vi "Target.vi"() -> ()   [LabVIEW 2019]
uses:
  <vilib>/rvi/DataTransferAndStorage/Container/Common/niFpgaContainerExecOnDevCompGetState.vi
  <vilib>/rvi/Emulation/niFpgaEmulationIsFPGAContextNoSignature.vi
  <vilib>/rvi/Emulation/niFpgaSctlEmulationGetInTimedLoop.vi
  <vilib>/rvi/errors/niFpgaSetErrorForExecOnDevCompSimple.vi
  <vilib>/rvi/eio/common/nirviEmuReportErrorAndStop.vi
  <vilib>/rvi/DataTransferAndStorage/Container/Common/niFpgaContainerGetUniqueNameForEmu.vi
  <vilib>/rvi/FIFO/Fifo_Resource/nirvififoEmulationSetSize.vi
  <vilib>/rvi/FIFO/Fifo_Resource/nirviFifoEmulationQueueMgr.vi
  <instcachedir>/0/nirviFifoEmulationQueueMgr_E5CAEC123FF24DC58D834DCA3CDAA9B5.lvgen/nirviFifoEmulationQueueMgr_E5CAEC123FF24DC58D834DCA3CDAA9B5_006.vi
  <vilib>/rvi/FIFO/Fifo_Resource/nirvififoEmulationDetermineInputValidOut.vi
  <vilib>/rvi/FIFO/Fifo_Resource/nirvififoEmulationCreateLock.vi
  <vilib>/rvi/Emulation/niFpgaProcessEmulError.vi
  <vilib>/rvi/FIFO/Fifo_Resource/nirvififoEmulationObtainLock.vi
  <vilib>/rvi/FIFO/Fifo_Resource/nirvififoEmulationReleaseLock.vi
  <vilib>/rvi/occurrence/nirviWaitOnOccurrenceBase.vi
  <vilib>/rvi/errors/nirviReportUnexpectedCaseInternalError.vi
  <vilib>/rvi/errors/nirviReportUnexpectedCaseInternalError (U32).vi
  <vilib>/Utility/error.llb/Clear Errors.vi
  <vilib>/rvi/interface/RandomDataEmulation/niFpgaRandomDataHandleErrors.vi
  <vilib>/rvi/DataTransferAndStorage/Container/XNode/niFpgaContainer.xnode
  <vilib>/rvi/FIFO/Fifo_Resource/niFpgaFifoEmulationRefIn.vi
panel:
  out "T5":u32 caption="Tick Count(mSec)"
  out "T4":u32 caption="Tick Count(mSec)"
  out "T3":u32 caption="Tick Count(mSec)"
  out "T2":u32 caption="Tick Count(mSec)"
  out "T1":u32 caption="Tick Count(mSec)"
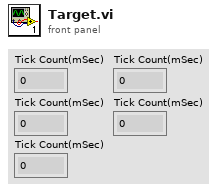
[diagram p1: front panel]
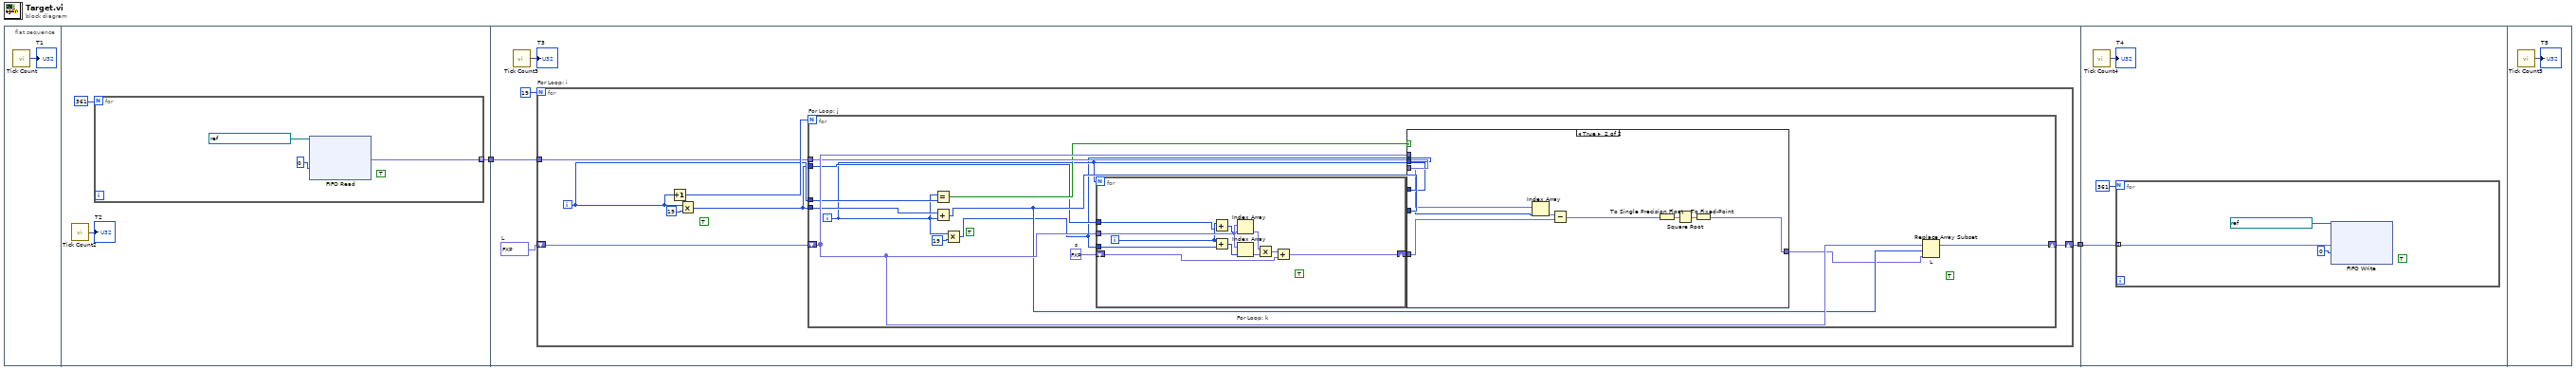
[diagram p0: block diagram]
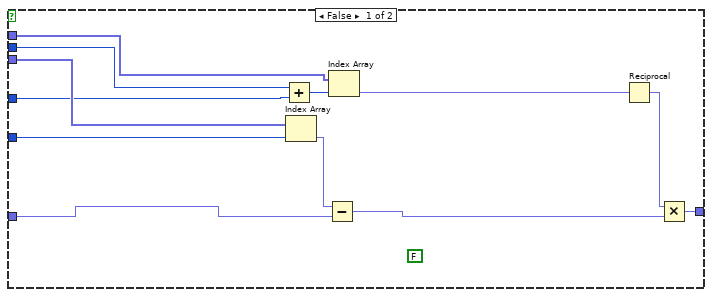
[diagram p2: hidden frame]
diagram:
  n1 = flat-sequence {
    tunnel: [w5] -> w2
    tunnel: w2 -> [w14]
    tunnel: [w13] -> w1
    tunnel: w1 -> [w68]
    frame #0 {
      n2 = call "Tick Count"() -> ("Tick Count(Ticks)"=→"T1":u32)
    }
    frame #1 {
      n3 = call "Tick Count2"() -> ("Tick Count(mSec)"=→"T2":u32)
      n4 = for {
        N: 361 -> [_]
        tunnel: [w9] -> w5 mode=indexing
        (unwired) TRUE
        n5 = xnode ("FIFO Read")("Timeout"=0, "FIFO In"=refnum<k21> "FIFO-host-to-Cholesky") -> ("Element"=w9:fxp<+/-,32,0>)  [unwired: 2 out]
      }
    }
    frame #2 {
      w12 = fxp<+,1,1>[] [0.0, 0.0, 0.0, 0.0, 0.0, 0.0, 0.0, 0.0, 0.0, 0.0, 0.0, 0.0, 0.0, 0.0, 0.0, 0.0, 0.0, 0.0, 0.0, 0.0, 0.0, 0.0, 0.0, 0.0, 0.0, 0.0, 0.0, 0.0, 0.0, 0.0, 0.0, 0.0, 0.0, 0.0, 0.0, 0.0, 0.0, 0.0, 0.0, 0.0, 0.0, 0.0, 0.0, 0.0, 0.0, 0.0, 0.0, 0.0, 0.0, 0.0, 0.0, 0.0, 0.0, 0.0, 0.0, 0.0, 0.0, 0.0, 0.0, 0.0, 0.0, 0.0, 0.0, 0.0, 0.0, 0.0, 0.0, 0.0, 0.0, 0.0, 0.0, 0.0, 0.0, 0.0, 0.0, 0.0, 0.0, 0.0, 0.0, 0.0, 0.0, 0.0, 0.0, 0.0, 0.0, 0.0, 0.0, 0.0, 0.0, 0.0, 0.0, 0.0, 0.0, 0.0, 0.0, 0.0, 0.0, 0.0, 0.0, 0.0, 0.0, 0.0, 0.0, 0.0, 0.0, 0.0, 0.0, 0.0, 0.0, 0.0, 0.0, 0.0, 0.0, 0.0, 0.0, 0.0, 0.0, 0.0, 0.0, 0.0, 0.0, 0.0, 0.0, 0.0, 0.0, 0.0, 0.0, 0.0, 0.0, 0.0, 0.0, 0.0, 0.0, 0.0, 0.0, 0.0, 0.0, 0.0, 0.0, 0.0, 0.0, 0.0, 0.0, 0.0, 0.0, 0.0, 0.0, 0.0, 0.0, 0.0, 0.0, 0.0, 0.0, 0.0, 0.0, 0.0, 0.0, 0.0, 0.0, 0.0, 0.0, 0.0, 0.0, 0.0, 0.0, 0.0, 0.0, 0.0, 0.0, 0.0, 0.0, 0.0, 0.0, 0.0, 0.0, 0.0, 0.0, 0.0, 0.0, 0.0, 0.0, 0.0, 0.0, 0.0, 0.0, 0.0, 0.0, 0.0, 0.0, 0.0, 0.0, 0.0, 0.0, 0.0, 0.0, 0.0, 0.0, 0.0, 0.0, 0.0, 0.0, 0.0, 0.0, 0.0, 0.0, 0.0, 0.0, 0.0, 0.0, 0.0, 0.0, 0.0, 0.0, 0.0, 0.0, 0.0, 0.0, 0.0, 0.0, 0.0, 0.0, 0.0, 0.0, 0.0, 0.0, 0.0, 0.0, 0.0, 0.0, 0.0, 0.0, 0.0, 0.0, 0.0, 0.0, 0.0, 0.0, 0.0, 0.0, 0.0, 0.0, 0.0, 0.0, 0.0, 0.0, 0.0, 0.0, 0.0, 0.0, 0.0, 0.0, 0.0, 0.0, 0.0, 0.0, 0.0, 0.0, 0.0, 0.0, 0.0, 0.0, 0.0, 0.0, 0.0, 0.0, 0.0, 0.0, 0.0, 0.0, 0.0, 0.0, 0.0, 0.0, 0.0, 0.0, 0.0, 0.0, 0.0, 0.0, 0.0, 0.0, 0.0, 0.0, 0.0, 0.0, 0.0, 0.0, 0.0, 0.0, 0.0, 0.0, 0.0, 0.0, 0.0, 0.0, 0.0, 0.0, 0.0, 0.0, 0.0, 0.0, 0.0, 0.0, 0.0, 0.0, 0.0, 0.0, 0.0, 0.0, 0.0, 0.0, 0.0, 0.0, 0.0, 0.0, 0.0, 0.0, 0.0, 0.0, 0.0, 0.0, 0.0, 0.0, 0.0, 0.0, 0.0, 0.0, 0.0, 0.0, 0.0, 0.0, 0.0, 0.0, 0.0, 0.0, 0.0, 0.0, 0.0, 0.0, 0.0, 0.0, 0.0, 0.0, 0.0, 0.0, 0.0, 0.0, 0.0, 0.0, 0.0, 0.0, 0.0, 0.0, 0.0, 0.0, 0.0, 0.0, 0.0, 0.0, 0.0, 0.0]  # L
      n6 = call "Tick Count3"() -> ("Tick Count(Ticks)"=→"T3":u32)
      n7 = for "For Loop: i" {
        N: 19 -> [_]
        shift-right: [w19] -> w13
        shift-left: w12 -> [w21]
        tunnel: w14 -> [w18]
        i -> [w17]
        (unwired) TRUE
        n8 = Increment(x=w17) -> (x+1=w20:i32)
        n9 = Multiply(x=w17, y=19) -> (x*y=w16:i32)
        n10 = for "For Loop: j" {
          N: w20 -> [_]
          tunnel: w17 -> [w31]
          shift-right: [w33] -> w19
          shift-left: w21 -> [w32]
          tunnel: w18 -> [w30]
          tunnel: w16 -> [w27]
          tunnel: w16 -> [w26]
          i -> [w25]
          (unwired) TRUE
          (unwired) TRUE
          w35 = fxp<+,1,1> 0.0  # s
          n11 = Equal?(x=w25, y=w31) -> (x = y?=w29:bool)
          n12 = Add(x=w27, y=w25) -> (x+y=w28:i32)
          n13 = Multiply(x=w25, y=19) -> (x*y=w24:i32)
          n14 = for "For Loop: k" {
            N: w25 -> [_]
            tunnel: w32 -> [w66]
            shift-right: [w64] -> w34
            shift-left: w35 -> [w65]
            tunnel: w26 -> [w62]
            tunnel: w24 -> [w61]
            i -> [w63]
            (unwired) TRUE
            n15 = Add(x=w63, y=w62) -> (x+y=w57:i32)
            n16 = Add(x=w63, y=w61) -> (x+y=w56:i32)
            n17 = Index Array(array=w66, index=w57) -> (element=w60:fxp<+,1,1>)
            n18 = Index Array(array=w66, index=w56) -> (element=w59:fxp<+,1,1>)
            n19 = Multiply(x=w60, y=w59) -> (x*y=w58:fxp<+,1,1>)
            n20 = Add(x=w58, y=w65) -> (x+y=w64:fxp<+,1,1>)
          }
          n21 = case shown="True" w29 {
            tunnel: w34 -> [w39 w55]
            tunnel: w32 -> [w47 _]
            tunnel: w30 -> [w44 w54]
            tunnel: w28 -> [w43 w53]
            tunnel: w25 -> [w42 _]
            tunnel: w24 -> [w41 _]
            tunnel: [w40 w52] -> w23
            frame False {
              (unwired) FALSE
              n22 = Add(x=w41, y=w42) -> (x+y=w37:i32)
              n23 = Index Array(array=w44, index=w43) -> (element=w36:fxp<+/-,32,0>)
              n24 = Subtract(x=w36, y=w39) -> (x-y=w38:fxp<+/-,32,0>)
              n25 = Index Array(array=w47, index=w37) -> (element=w46:fxp<+,1,1>)
              n26 = Reciprocal(x=w46) -> (1/x=w45:fxp<+,2,1>)
              n27 = Multiply(x=w45, y=w38) -> (x*y=w40:fxp<+/-,33,0>)
            }
            frame True {
              n28 = Index Array(array=w54, index=w53) -> (element=w48:fxp<+/-,32,0>)
              n29 = Subtract(x=w48, y=w55) -> (x-y=w50:fxp<+/-,32,0>)
              n30 = To Single Precision Float(number=w50) -> (single precision float=w49:sgl)
              n31 = Square Root(x=w49) -> (sqrt(x)=w51:sgl)
              n32 = To Fixed-Point(number=w51) -> (fixed-point=w52:fxp<+/-,32,16>)  [unwired: 1 in]
            }
          }
          n33 = Replace Array Subset "L"(array=w32, new element=w23, index=w28) -> (w33:fxp<+,1,1>[])
        }
      }
    }
    frame #3 {
      n34 = call "Tick Count4"() -> ("Tick Count(Ticks)"=→"T4":u32)
      n35 = for {
        N: 361 -> [_]
        tunnel: w68 -> [w72] mode=indexing
        (unwired) TRUE
        n36 = xnode ("FIFO Write")("Element"=w72, "Timeout"=0, "FIFO In"=refnum<k21> "FIFO-Cholesky-to-host") -> ()  [unwired: 2 out]
      }
    }
    frame #4 {
      n37 = call "Tick Count5"() -> ("Tick Count(Ticks)"=→"T5":u32)
    }
  }
